vi "생산자 소비자.vi"() -> ()   [LabVIEW 2014]
panel:
  in  "메시지 큐 삭제":bool
  in  "EMG 메시지":bool
  in  "메시지":string[](array[string])
  in  "Send":bool
  out "원소":string
  in  "정지":bool
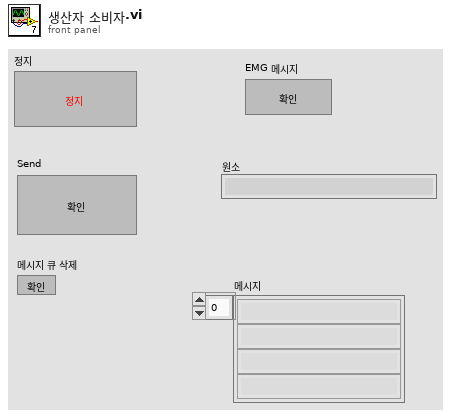
[diagram p1: front panel]
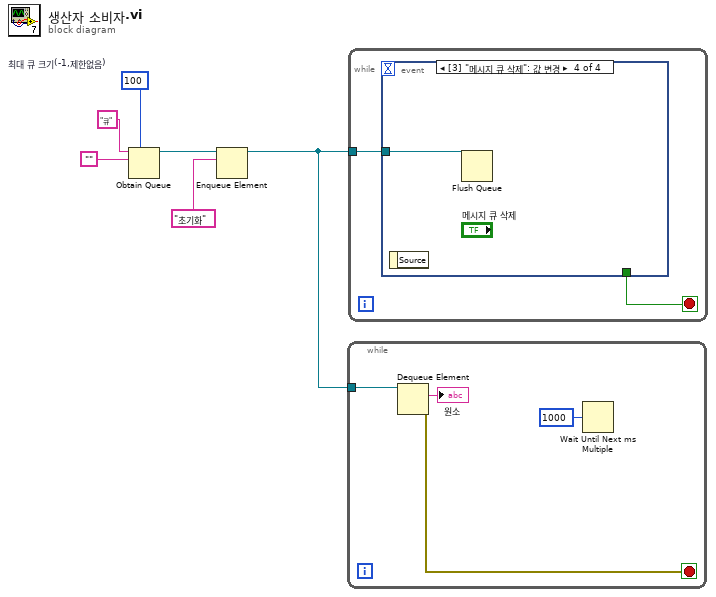
[diagram p0: block diagram]
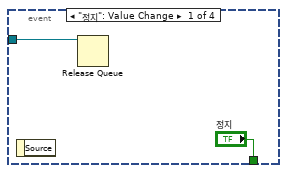
[diagram p2: hidden frame]
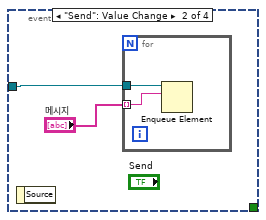
[diagram p3: hidden frame]
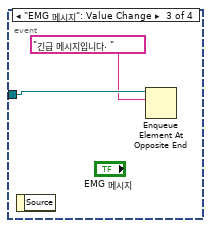
[diagram p4: hidden frame]
diagram:
  w2 = 100  # 최대 큐 크기(-1,제한없음)
  n1 = Obtain Queue(max queue size (-1, unlimited)=w2, name (unnamed)="큐" ("이름(이름없음)"), element data type="") -> (queue out=w6:refnum<queue>)  [unwired: 2 in, 2 out]
  n2 = Enqueue Element(queue=w6, element="초기화") -> (queue out=w1:refnum<queue>)  [unwired: 2 in, 2 out]
  n3 = while {
    tunnel: w1 -> [w10]
    stop <- w8 stop-if-true
    n4 = Dequeue Element(queue=w10) -> (element=→"원소":string, error out=w8:errorcluster)  [unwired: 2 in, 2 out]
    n5 = Wait Until Next ms Multiple(millisecond multiple=u32 1000 ("ms 배수")) -> ()  [unwired: 1 out]
  }
  n6 = while {
    tunnel: w1 -> [w11]
    stop <- w12 stop-if-true
    n7 = event shown="[3] \"메시지 큐 삭제\": 값 변경" {
      selector: _ -> [_ _ _ _]
      dyn-events: _ -> [_ _ _ _]
      timeout: _ -> [_ _ _ _]
      tunnel: ["정지" _ _ _] -> w12
      tunnel: w11 -> [w13 w16 w20 w21]
      event "정지": Value Change {
        n8 = event-data() -> ()  [unwired: 1 in, 1 out]
        n9 = Release Queue(queue=w13) -> ()  [unwired: 2 in, 3 out]
      }
      event "Send": Value Change {
        n10 = event-data() -> ()  [unwired: 1 in, 1 out]
        n11 = for {
          tunnel: w16 -> [w18]
          tunnel: "메시지" -> [w17] mode=indexing
          n12 = Enqueue Element(queue=w18, element=w17) -> ()  [unwired: 2 in, 3 out]
        }
      }
      event "EMG 메시지": Value Change {
        n13 = event-data() -> ()  [unwired: 1 in, 1 out]
        n14 = Enqueue Element At Opposite End(queue=w20, element="긴급 메시지입니다. " ("원소")) -> ()  [unwired: 2 in, 3 out]
      }
      event "메시지 큐 삭제": Value Change {
        n15 = event-data() -> ()  [unwired: 1 in, 1 out]
        n16 = Flush Queue(queue=w21) -> ()  [unwired: 1 in, 3 out]
      }
    }
  }
